vi "SubHid_Generator.vi"(1 "Generator signal type":string(combo), 2 "Amplitude":dbl, 3 "Gfreq":dbl=10.0 format="%0.4e", 4 "task/channels in":refnum<k21>) -> (0 "Przebiegi generatora":dbl[][](graph))   [LabVIEW 2020]
uses:
  <vilib>/Analysis/3filter.llb/Filter Passband Type.ctl
  <vilib>/DAQmx/write.llb/DAQmx Write (Analog 2D DBL NChan NSamp).vi
  <vilib>/Analysis/3filter.llb/Butterworth Filter (DBL).vi
  <vilib>/DAQmx/configure/timing.llb/DAQmx Timing (Sample Clock).vi
  <vilib>/DAQmx/miscellaneous.llb/DAQmx Fill In Error Info.vi
  <vilib>/Analysis/NI_AALBase.lvlib
  <resource>/objmgr/daqmx.rc
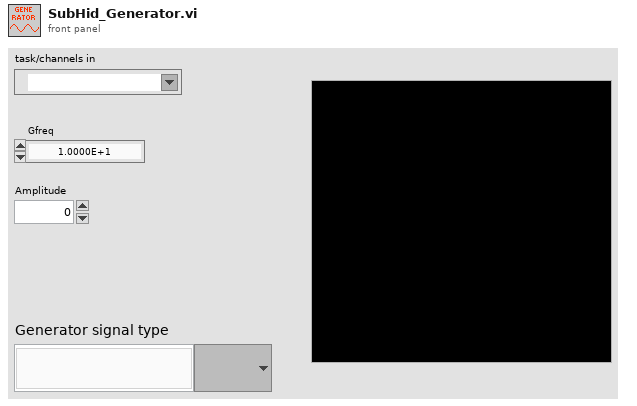
[diagram p1: front panel]
types:
  T1 = typedef "NI_AALBase.lvlib/Filter Passband Type.ctl" = enum32{"Lowpass", "Highpass", "Bandpass", "Bandstop"}
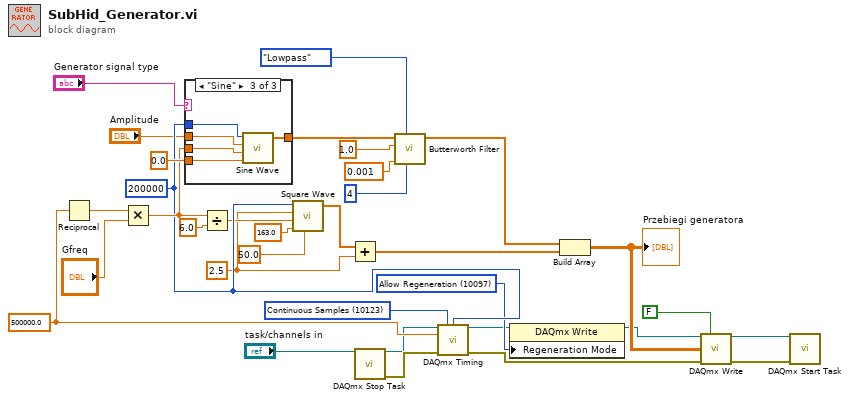
[diagram p0: block diagram]
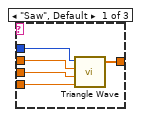
[diagram p2: hidden frame]
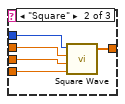
[diagram p3: hidden frame]
diagram:
  w29 = 200000 ("Gsamples")
  w2 = 2.5 ("amplitude")
  w33 = 500000.0 ("x")
  w11 = 10097 items=["Allow Regeneration"=10097, "Do Not Allow Regeneration"=10158] ("RegenMode")
  w8 = 10123 items=["Finite Samples"=10178, "Continuous Samples"=10123, "Hardware Timed Single Point"=12522] ("sample mode")
  n1 = Reciprocal(x=w33) -> (1/x=w21:dbl)
  n2 = Multiply(x=w21, y="Gfreq") -> (x*y=w30:dbl)
  n3 = case shown="\"Sine\"" "Generator signal type" {
    tunnel: w29 -> [w34 w43 w44]
    tunnel: w30 -> [w38 w41 w46]
    tunnel: 0.0 ("phase in") -> [w37 w40 w45]
    tunnel: [w36 w39 w48] -> w32
    tunnel: "Amplitude" -> [w35 w42 w47]
    frame "Saw", Default {
      n4 = call <vilib>:"Triangle Wave.vi"("samples"=w34, "amplitude"=w35, "frequency"=w38, "phase in"=w37) -> ("triangle wave"=w36:dbl[])  [unwired: 1 in, 2 out]
    }
    frame "Square" {
      n5 = call <vilib>:"Square Wave.vi"("samples"=w43, "amplitude"=w42, "frequency"=w41, "phase in"=w40) -> ("square wave"=w39:dbl[])  [unwired: 2 in, 2 out]
    }
    frame "Sine" {
      n6 = call <vilib>:"Sine Wave.vi"("samples"=w44, "amplitude"=w47, "frequency"=w46, "phase in"=w45) -> ("sine wave"=w48:dbl[])  [unwired: 1 in, 2 out]
    }
  }
  n7 = Divide(x=w30, y=6.0) -> (x/y=w26:dbl)
  n8 = call <vilib>:"Square Wave.vi"("samples"=w29, "amplitude"=w2, "frequency"=w26, "duty cycle (%)"=50.0, "phase in"=163.0) -> ("square wave"=w18:dbl[])  [unwired: 1 in, 2 out]
  n9 = Add(x=w18, y=w2) -> (x+y=w19:dbl[])
  n10 = call <vilib>:"DAQmx Stop Task.vi"("task/channels in"="task/channels in") -> ("task out"=w15:refnum<k21>, "error out"=w16:errorcluster)  [unwired: 13 in]
  n11 = call-poly <vilib>:"Butterworth Filter.vi"("order"=4, "filter type"=Filter_Passband_Type."Lowpass", "low cutoff freq: fl"=0.001, "sampling freq: fs"=1.0, "X"=w32) -> ("Filtered X"=w28:dbl[])  [unwired: 3 in, 1 out]
  n12 = call-poly <vilib>:"DAQmx Timing.vi"("task/channels in"=w15, "sample mode"=w8, "samples per channel"=w29, "rate"=w33, "error in"=w16) -> ("task out"=w9:refnum<k21>, "error out"=w1:errorcluster)  [unwired: 9 in]
  n13 = property class="DAQmx Write"(reference=w9, "Regeneration Mode"=w11) -> (reference out=w10:refnum<k21>)  [unwired: 1 in, 1 out]
  n14 = Build Array(w28, w19) -> (w27:dbl[][])
  "Przebiegi generatora" <- w27
  n15 = call-poly <vilib>:"DAQmx Write.vi"("task/channels in"=w10, "auto start"=FALSE, "data"=w27, "error in"=w1) -> ("task out"=w13:refnum<k21>, "error out"=w14:errorcluster)  [unwired: 9 in, 1 out]
  n16 = call <vilib>:"DAQmx Start Task.vi"("task/channels in"=w13, "error in"=w14) -> ()  [unwired: 12 in, 2 out]
